vi "BUILD ARRAY vf.vi"(11 "data":string[][](array[string])) -> (3 "Array":bool[][][](array[boolean]))   [LabVIEW 2019]
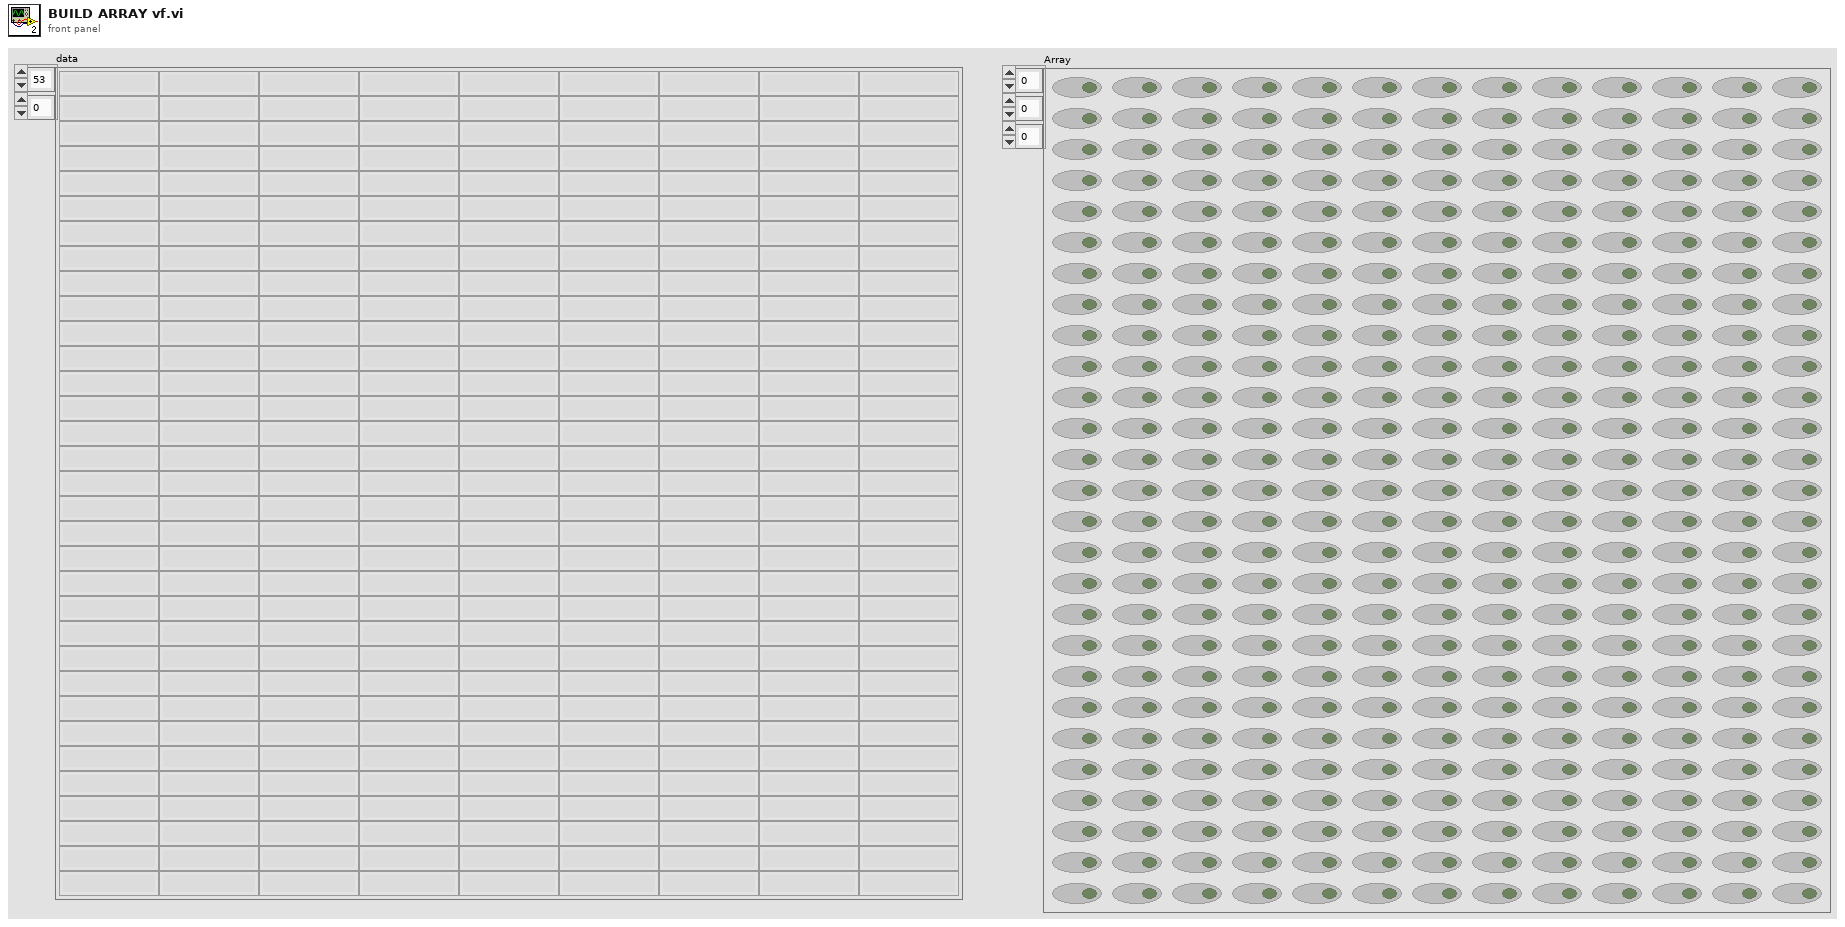
[diagram p1: front panel]
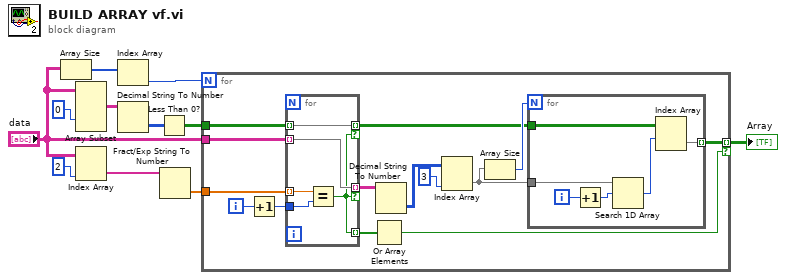
[diagram p0: block diagram]
diagram:
  n1 = Array Size(array="data") -> (size(s)=w3:i32[])
  n2 = Array Subset(array="data", index (col)=0 ("index")) -> (w5:string[][])  [unwired: 3 in]
  n3 = Index Array(array="data", index (col)=2 ("disabled index (col)")) -> (element=w8:string[])  [unwired: 1 in]
  n4 = Index Array(array=w3) -> (element=w2:i32)  [unwired: 1 in]
  n5 = Decimal String To Number(string=w5) -> (number=w6:i32[][])  [unwired: 2 in, 1 out]
  n6 = Less Than 0?(x=w6) -> (x < 0?=w10:bool[][])
  n7 = Fract/Exp String To Number(string=w8) -> (number=w9:dbl[])  [unwired: 3 in, 1 out]
  n8 = for {
    N: w2 -> [_]
    tunnel: w9 -> [w25]
    tunnel: w10 -> [w24]
    tunnel: [w18] -> w11 mode=indexing if=w12
    tunnel: "data" -> [w17]
    i -> [w23]
    n9 = Increment(x=w23) -> (x+1=w22:i32)
    n10 = for {
      tunnel: w25 -> [w36] mode=indexing
      tunnel: w22 -> [w35]
      tunnel: w24 -> [w34] mode=indexing
      tunnel: [w34] -> w19 mode=indexing if=w32
      tunnel: [w33] -> w16 mode=indexing if=w32
      tunnel: w17 -> [w33] mode=indexing
      tunnel: [w32] -> w13 mode=indexing
      n11 = Equal?(x=w36, y=w35) -> (x = y?=w32:bool)
    }
    n12 = Or Array Elements(Boolean array=w13) -> (logical OR=w12:bool)
    n13 = Decimal String To Number(string=w16) -> (number=w15:i32[][])  [unwired: 2 in, 1 out]
    n14 = Index Array(array=w15, index (col)=3 ("disabled index (col)")) -> (element=w14:i32[])  [unwired: 1 in]
    n15 = Array Size(array=w14) -> (size(s)=w21:i32)
    n16 = for {
      N: w21 -> [_]
      tunnel: w14 -> [w31]
      tunnel: w19 -> [w28]
      tunnel: [w26] -> w18 mode=indexing
      i -> [w30]
      n17 = Increment(x=w30) -> (x+1=w29:i32)
      n18 = Search 1D Array(1D array=w31, element=w29) -> (index of element=w27:i32)  [unwired: 1 in]
      n19 = Index Array(array=w28, index (row)=w27) -> (element=w26:bool[])  [unwired: 1 in]
    }
  }
  "Array" <- w11
